vi "ledip.vi"() -> ()   [LabVIEW 2016]
uses:
  <vilib>/LabVIEW Interface for Arduino/Type Defs/Pin Mode.ctl
  <vilib>/LabVIEW Interface for Arduino/LabVIEW Interface for Arduino.lvlib
panel:
  out "Numeric":dbl format="%#_13g"
  in  "Analog Input Pin (0)":u8
  out "Gauge":dbl(knob) scale=0.0..10.0
  out "Thermometer":dbl(slide) scale=0.0..100.0
  in  "stop":bool
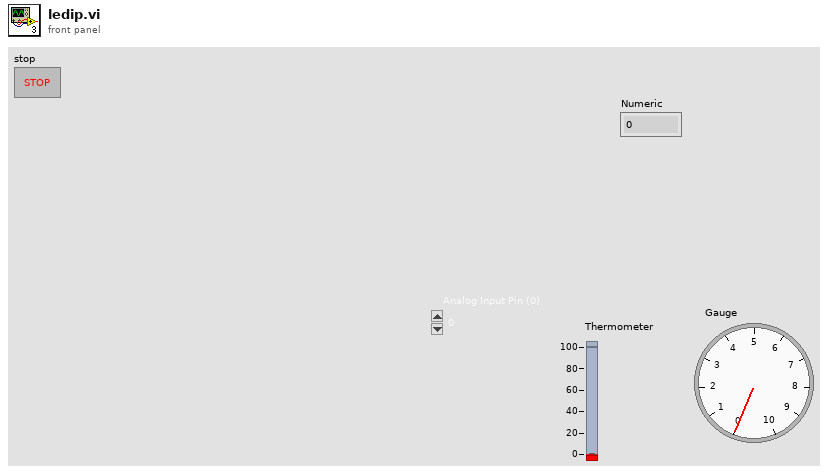
[diagram p1: front panel]
types:
  T1 = typedef "LabVIEW Interface for Arduino.lvlib/Pin Mode.ctl" = enum8{"Input", "Output"}
  T2 = typedef "LabVIEW Interface for Arduino.lvlib/Arduino Resource.ctl" = cluster{"VISA resource":refnum<visa-resource-name>, "Board Type":T3, "Connection Type":enum8{"USB / Serial"}, "Bytes Per Packet (15)":u8}
  T3 = typedef "LabVIEW Interface for Arduino.lvlib/Board Type.ctl" = enum16{"Uno", "Dimuelanove w/Atmega 328", "Mega 2560"}
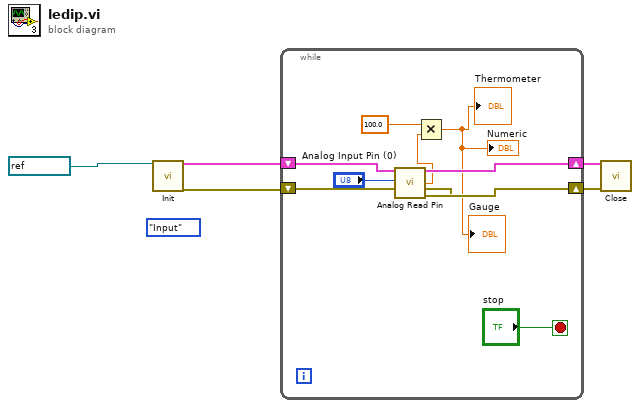
[diagram p0: block diagram]
diagram:
  (unwired) Pin_Mode."Input" ("Pin Mode (Input)")
  n1 = call <vilib>:"Init.vi"("VISA resource"=refnum<visa-resource-name> "COM3") -> ("Arduino Resource"=w1:T2, "error out"=w2:errorcluster)  [unwired: 17 in]
  n2 = while {
    shift-right: [w14] -> w5
    shift-left: w1 -> [w11]
    shift-right: [w13] -> w4
    shift-left: w2 -> [w10]
    stop <- "stop" stop-if-true
    n3 = call <vilib>:"Analog Read Pin.vi"("Arduino Resource"=w11, "Analog Input Pin (0)"="Analog Input Pin (0)", "error in"=w10) -> ("Arduino Resource"=w14:T2, "Voltage"=w7:dbl, "error out"=w13:errorcluster)  [unwired: 10 in]
    n4 = Multiply(x=100.0, y=w7) -> (x*y=→"Thermometer" →"Gauge" →"Numeric":dbl)
  }
  n5 = call <vilib>:"Close.vi"("Arduino Resource"=w5, "error in"=w4) -> ()  [unwired: 13 in, 1 out]
